vi "DeltaAngle_Degrees.vi"(1 "EndAngle (deg)":dbl, 2 "StartAngle (deg)":dbl) -> (0 "DeltaAngle (deg)":dbl)   [LabVIEW 2017]
uses:
  45e4bb04-65c6-42ed-a146-56a661e49e85.vi
panel:
  # "Computes shortest angle change necessary to go from\nStartAngle degrees to EndAngle degrees\nHandles angles with range [0,360] or [-180,180]"
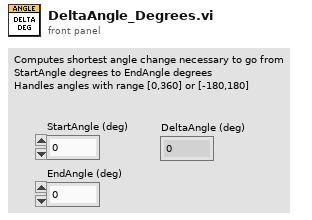
[diagram p1: front panel]
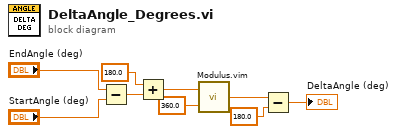
[diagram p0: block diagram]
diagram:
  n1 = Subtract(x="EndAngle (deg)", y="StartAngle (deg)") -> (x-y=w6:dbl)
  n2 = Add(x=180.0, y=w6) -> (x+y=w5:dbl)
  n3 = call "Modulus.vim"("y"=360.0, "x"=w5) -> ("x%y"=w3:dbl)
  n4 = Subtract(x=w3, y=180.0) -> (x-y=→"DeltaAngle (deg)":dbl)
